vi "Copy Template Library.vi"(7 "App":refnum<vi>, 8 "error in (no error)":errorcluster, 10 "Destination lvlib Path":path=path "C:/dev/proto/hello/lv/MyTest/MyTest.lvlib", 11 "Source lvlib Path":path=path "C:/dev/lv20CE/lv-protoc/Enum Template/Enum Template.lvlib") -> (0 "error out":errorcluster, 1 "Nested Libraries":refnum<vi>[](array[refnum]), 2 "VIs":refnum<vi>[](array[refnum]), 3 "Library":refnum<vi>)   [LabVIEW 2020, in "LV-Protoc.lvlib"]
uses:
  LV-Protoc.lvlib
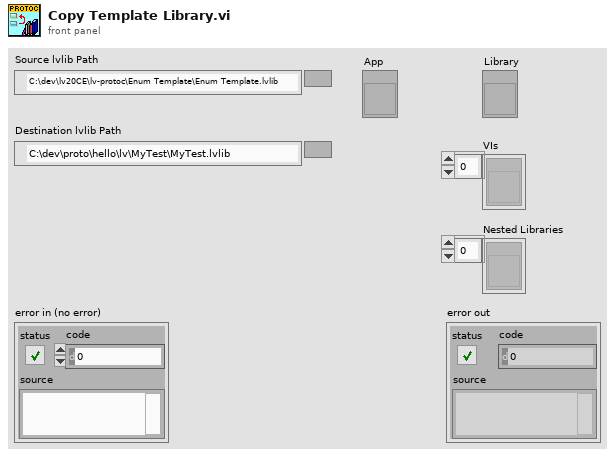
[diagram p1: front panel]
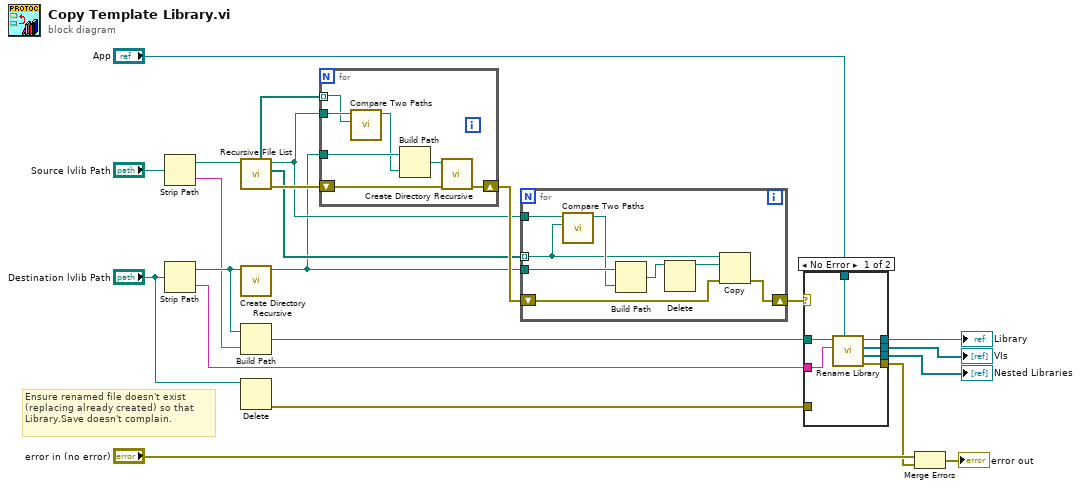
[diagram p0: block diagram]
diagram:
  # "Ensure renamed file doesn't exist (replacing already created) so that Library.Save doesn't complain."
  n1 = Strip Path(path="Source lvlib Path") -> (stripped path=w15:path, name=w19:string)
  n2 = Strip Path(path="Destination lvlib Path") -> (stripped path=w20:path, name=w14:string)
  n3 = call <vilib>:"Recursive File List.vi"("Folder Path"=w15) -> ("error out"=w22:errorcluster, "All Files in Dir"=w8:path[], "dup Folder Path"=w7:path, "All Folders"=w10:path[])  [unwired: 6 in, 1 out]
  n4 = call <vilib>:"Create Directory Recursive.vi"("directory"=w20) -> ("directory copy"=w6:path)  [unwired: 4 in, 2 out]
  n5 = Build Path(base path=w20, name or relative path=w19) -> (appended path=w13:path)
  n6 = Delete(path (use dialog)="Destination lvlib Path") -> (error out=w12:errorcluster)  [unwired: 4 in, 2 out]
  n7 = for {
    tunnel: w7 -> [w29]
    tunnel: w10 -> [w28] mode=indexing
    tunnel: w6 -> [w27]
    shift-right: [w24] -> w9
    shift-left: w22 -> [w23]
    n8 = call <vilib>:"Compare Two Paths.vi"("Path 2"=w28, "Path 1"=w29) -> ("Relative Path from 1 to 2"=w26:path)  [unwired: 6 in, 3 out]
    n9 = Build Path(base path=w27, name or relative path=w26) -> (appended path=w25:path)
    n10 = call <vilib>:"Create Directory Recursive.vi"("error in (no error)"=w23, "directory"=w25) -> ("error out"=w24:errorcluster)  [unwired: 3 in, 2 out]
  }
  n11 = for {
    shift-right: [w30] -> w5
    shift-left: w9 -> [w37]
    tunnel: w8 -> [w32] mode=indexing
    tunnel: w7 -> [w36]
    tunnel: w6 -> [w35]
    n12 = call <vilib>:"Compare Two Paths.vi"("Path 2"=w32, "Path 1"=w36) -> ("Relative Path from 1 to 2"=w34:path)  [unwired: 6 in, 3 out]
    n13 = Build Path(base path=w35, name or relative path=w34) -> (appended path=w33:path)
    n14 = Delete(path (use dialog)=w33) -> (deleted path=w31:path)  [unwired: 4 in, 2 out]
    n15 = Copy(8:w37, 10:w31, 11:w32) -> (0:w30:errorcluster)  [unwired: 2 in, 2 out]
  }
  n16 = case shown="No Error" w5 {
    selector: w5 -> [_ w45]
    tunnel: w14 -> [w43 _]
    tunnel: w13 -> [w44 _]
    tunnel: w12 -> [_ _]
    tunnel: [w42 w45] -> w11
    tunnel: "App" -> [w41 _]
    tunnel: [w40 _] -> w3
    tunnel: [w39 _] -> w2
    tunnel: [w38 _] -> w1
    frame No Error {
      n17 = call "Rename Library.vi"("App"=w41, "New Name"=w43, "Original Library"=w44) -> ("error out"=w42:errorcluster, "Nested Libraries"=w38:refnum<vi>[], "VIs"=w39:refnum<vi>[], "Library"=w40:refnum<vi>)  [unwired: 5 in]
    }
    frame Error {
    }
  }
  "Library" <- w3
  "VIs" <- w2
  "Nested Libraries" <- w1
  n18 = Merge Errors("error in (no error)", w11) -> (→"error out":errorcluster)
